vi "Test ServiceNET Bob.vi"() -> ()   [LabVIEW 2016]
uses:
  rqcBob Send Data/rqcBob ServiceNET Send Data U32.vi
panel:
  in  "Data":u32[](array[numeric])
  in  "Send data":bool
  out "error out":errorcluster
  out "connected?":bool
  in  "stop":bool
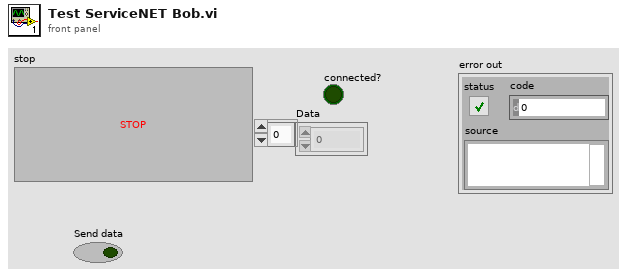
[diagram p1: front panel]
types:
  T1 = typedef "rqcBob ServiceNET control.ctl" = cluster{"connection ID":refnum<k5>, "connected?":bool, "Alice's IP address":string, "port":u16}
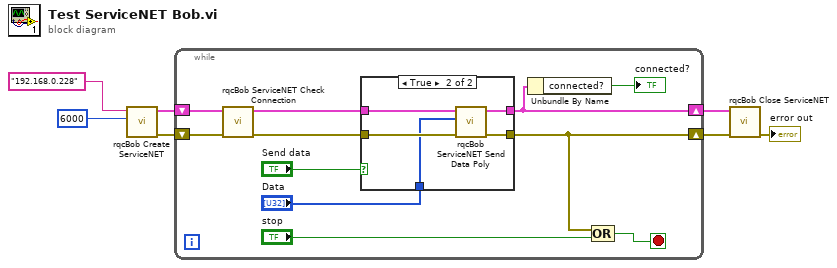
[diagram p0: block diagram]
diagram:
  n1 = call "rqcBob Create ServiceNET.vi"("port"=u16 6000, "Alice's IP address"="192.168.0.228") -> ("error out"=w4:errorcluster, "rqcBob ServiceNET control"=w5:T1)  [unwired: 8 in]
  n2 = while {
    shift-right: [w9] -> w3
    shift-left: w5 -> [w18]
    shift-right: [w11] -> w2
    shift-left: w4 -> [w17]
    stop <- w15 stop-if-true
    n3 = call "rqcBob ServiceNET Check Connection.vi"("error in"=w17, "rqcBob ServiceNET in"=w18) -> ("error out"=w12:errorcluster, "rqcBob ServiceNET out"=w13:T1)  [unwired: 8 in]
    n4 = case shown="True" "Send data" {
      tunnel: w13 -> [w20 w25]
      tunnel: [w20 w24] -> w9
      tunnel: w12 -> [w19 w22]
      tunnel: [w19 w23] -> w11
      tunnel: "Data" -> [_ w21]
      frame False {
      }
      frame True {
        n5 = call-poly "rqcBob ServiceNET Send Data Poly.vi"("error in"=w22, "Data"=w21, "rqcBob ServiceNET in"=w25) -> ("error out"=w23:errorcluster, "rqcBob ServiceNET out"=w24:T1)  [unwired: 7 in]
      }
    }
    n6 = Unbundle By Name(w9) -> ("connected?"=→"connected?":bool)
    n7 = Compound Arithmetic op=OR(w11, "stop") -> (w15:bool)
  }
  n8 = call "rqcBob Close ServiceNET.vi"("error in"=w2, "rqcBob ServiceNET control"=w3) -> ("error out"=→"error out":errorcluster)  [unwired: 9 in]
